vi "Close Ref.vi"(8 "error in (no error)":errorcluster, 11 "PXI 8513 in":refnum<class "PXI 8513.lvclass">) -> (0 "error out":errorcluster, 3 "PXI 8513 out":refnum<class "PXI 8513.lvclass">)   [LabVIEW 2021, in "CAN.lvlib" / "PXI 8513.lvclass"]
uses:
  PXI 8513.lvclass
  PXI 8513.lvclass/PXI 8513.ctl
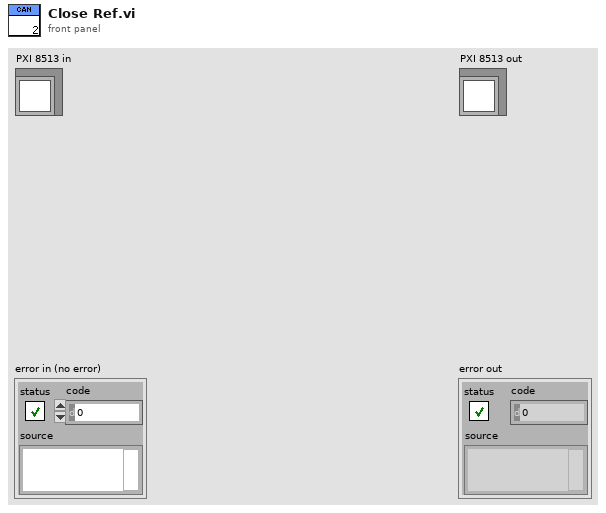
[diagram p1: front panel]
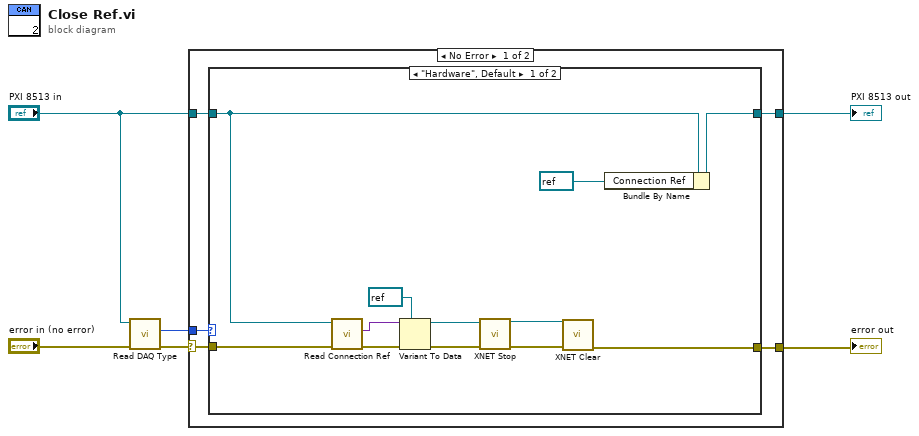
[diagram p0: block diagram]
diagram:
  n1 = call-dynamic "Read DAQ Type.vi"("error in (no error)"="error in (no error)", "PXI 8513 in"="PXI 8513 in") -> ("error out"=w5:errorcluster, "DAQ Type"=w4:enum16{"Hardware", "Simulation"})  [unwired: 7 in, 1 out]
  n2 = case shown="No Error" w5 {
    selector: w5 -> [w9 w26]
    tunnel: w4 -> [w11 _]
    tunnel: "PXI 8513 in" -> [w10 w27]
    tunnel: [w8 w26] -> w2
    tunnel: [w7 w27] -> w1
    frame No Error {
      n3 = case shown="\"Hardware\", Default" w11 {
        tunnel: w10 -> [w14 w25]
        tunnel: w9 -> [w23 w24]
        tunnel: [w15 w24] -> w8
        tunnel: [w13 w25] -> w7
        frame "Hardware", Default {
          n4 = call-dynamic "Read Connection Ref.vi"("error in (no error)"=w23, "PXI 8513 in"=w14) -> ("error out"=w21:errorcluster, "Connection Ref"=w20:variant)  [unwired: 7 in, 1 out]
          n5 = Variant To Data(error in=w21, type=refnum<k21> refnum ("session out"), Variant=w20) -> (data=w17:refnum<k21>, error out=w19:errorcluster)
          n6 = call <vilib>:"XNET Stop.vi"("session in"=w17, "error in (no error)"=w19) -> ("session out"=w16:refnum<k21>, "error out"=w18:errorcluster)  [unwired: 12 in]
          n7 = call <vilib>:"XNET Clear.vi"("session in"=w16, "error in (no error)"=w18) -> ("error out"=w15:errorcluster)  [unwired: 13 in]
          n8 = Bundle By Name(cluster=w14, "Connection Ref"=refnum<k21> refnum ("session out")) -> (w13:refnum<class "PXI 8513.lvclass">)
        }
        frame "Simulation" {
        }
      }
    }
    frame Error {
    }
  }
  "error out" <- w2
  "PXI 8513 out" <- w1
